vi "NEO Sensor Fault detection.vi"() -> (0 "Array":string[](array[string]), 1 "Cascade Sensor":bool, 2 "Rhino Sensors":bool, 3 "Drivebase Sensors":bool)   [LabVIEW 2018]
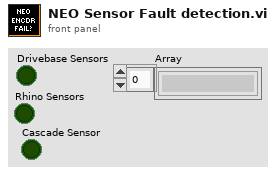
[diagram p1: front panel]
types:
  T1 = typedef "WPI_MotorControlDeviceRef.ctl" = cluster{"DeviceStatus":errorcluster, "Type":T2, "PWM":cluster{"PWM Channel":T3, "DeadBand":T4}, "CAN":cluster{"Device Number":u8, "SetOutput VI Ref":variant, "GetOutput VI Ref":variant, "Enable VI Ref":variant, "Disable VI Ref":variant, "Data":variant}, "Invert":bool, "DIO PWM":cluster{"PWM \"Enable\" Channel":T3, "DIOChannel":T5, "PWM Rate":dbl}}
  T2 = typedef "WPI_MotorControlType.ctl" = enum16{"PWM", "CAN", "DIO PWM"}
  T3 = typedef "FPGA_DIOPWMChannel.ctl" = enum8{"PWM 0", "PWM 1", "PWM 2", "PWM 3", "PWM 4", "PWM 5", "PWM 6", "PWM 7", "PWM 8", "PWM 9", "PWM MXP 0", "PWM MXP 1", "PWM MXP 2", "PWM MXP 3", "PWM MXP 4", "PWM MXP 5", "PWM MXP 6", "PWM MXP 7", "PWM MXP 8", "PWM MXP 9", "Invalid"}
  T4 = typedef "WPI_PWMDeadband.ctl" = cluster{"Name":string, "maxPositivePwm":i32, "minPositivePwm":i32, "centerPwm":i32, "maxNegativePwm":i32, "minNegativePwm":i32, "angularRange":u16}
  T5 = typedef "FPGA_DIOChannel.ctl" = enum8{"DIO 0", "DIO 1", "DIO 2", "DIO 3", "DIO 4", "DIO 5", "DIO 6", "DIO 7", "DIO 8", "DIO 9", "DIO MXP 0", "DIO MXP 1", "DIO MXP 2", "DIO MXP 3", "DIO MXP 4", "DIO MXP 5", "DIO MXP 6", "DIO MXP 7", "DIO MXP 8", "DIO MXP 9", "DIO MXP 10", "DIO MXP 11", "DIO MXP 12", "DIO MXP 13", "DIO MXP 14", "DIO MXP 15", "SPI Port CS1", "SPI Port CS2", "SPI Port CS3", "SPI Port MISO", "SPI Port MOSI", "Invalid"}
  T6 = typedef "Spark MAX Faults.ctl" = cluster{"Hard Limit Rev":bool, "Hard Limit Fwd":bool, "Soft Limit Fwd":bool, "Soft Limit Rev":bool, "Other Fault":bool, "DRV Fault":bool, "Has Reset?":bool, "CAN RX":bool, "CAN TX":bool, "EEPROM CRC":bool, "Stall":bool, "Sensor Fault":bool, "Motor Type Fault":bool, "IWDT Reset":bool, "Over Current":bool, "Brownout":bool}
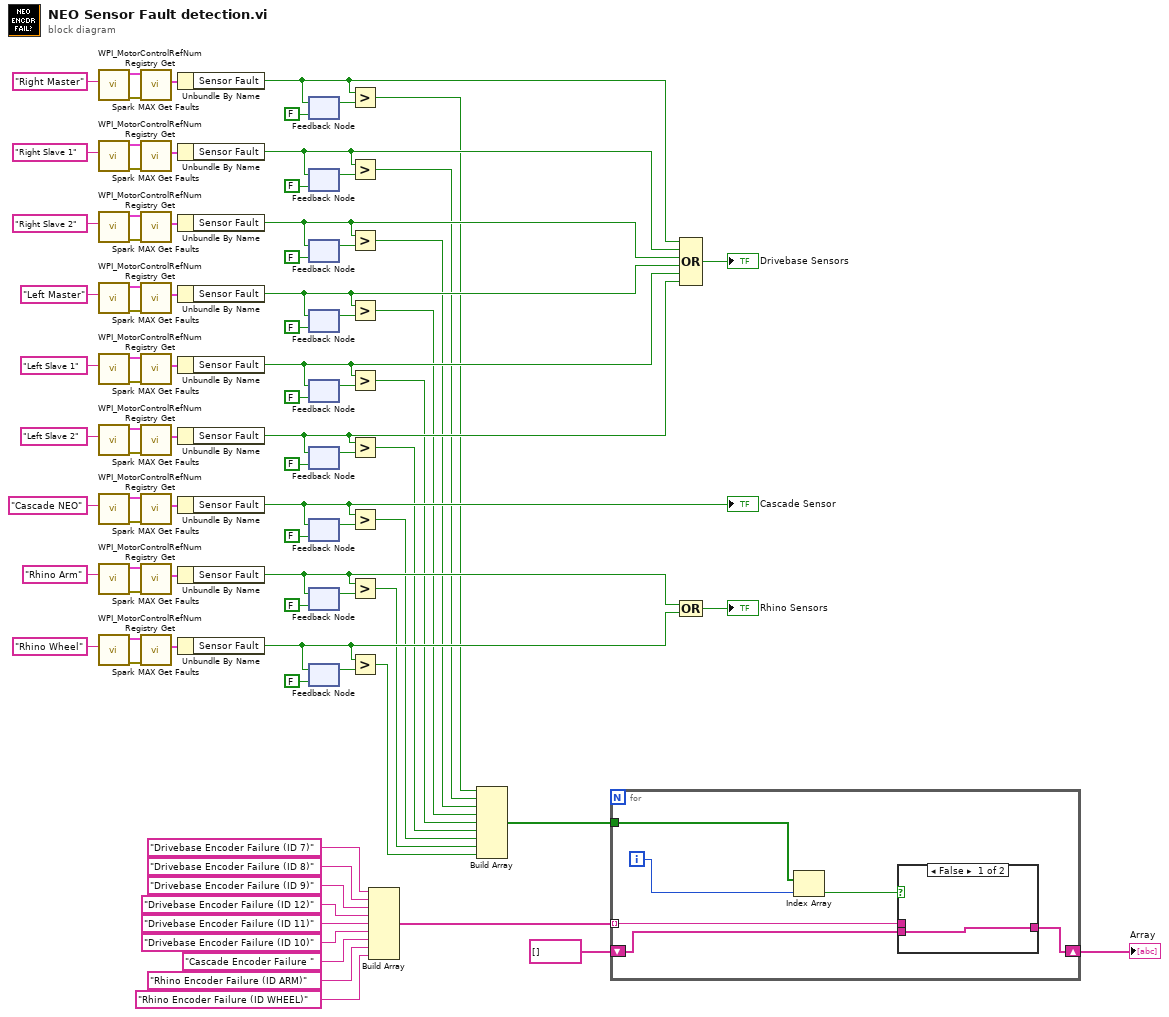
[diagram p0: block diagram]
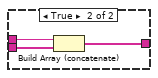
[diagram p2: hidden frame]
diagram:
  n1 = call <vilib>:"WPI_MotorControlRefNum Registry Get.vi"("refnum name"="Right Master") -> ("error out"=w75:errorcluster, "MotorControlDevRef"=w81:T1)  [unwired: 9 in]
  n2 = call <vilib>:"WPI_MotorControlRefNum Registry Get.vi"("refnum name"="Right Slave 1") -> ("error out"=w74:errorcluster, "MotorControlDevRef"=w80:T1)  [unwired: 9 in]
  n3 = call <vilib>:"WPI_MotorControlRefNum Registry Get.vi"("refnum name"="Right Slave 2") -> ("error out"=w73:errorcluster, "MotorControlDevRef"=w79:T1)  [unwired: 9 in]
  n4 = call <vilib>:"WPI_MotorControlRefNum Registry Get.vi"("refnum name"="Left Master") -> ("error out"=w72:errorcluster, "MotorControlDevRef"=w78:T1)  [unwired: 9 in]
  n5 = call <vilib>:"WPI_MotorControlRefNum Registry Get.vi"("refnum name"="Left Slave 1") -> ("error out"=w71:errorcluster, "MotorControlDevRef"=w77:T1)  [unwired: 9 in]
  n6 = call <vilib>:"WPI_MotorControlRefNum Registry Get.vi"("refnum name"="Left Slave 2") -> ("error out"=w70:errorcluster, "MotorControlDevRef"=w76:T1)  [unwired: 9 in]
  n7 = call <vilib>:"WPI_MotorControlRefNum Registry Get.vi"("refnum name"="Cascade NEO") -> ("error out"=w61:errorcluster, "MotorControlDevRef"=w60:T1)  [unwired: 9 in]
  n8 = call <vilib>:"WPI_MotorControlRefNum Registry Get.vi"("refnum name"="Rhino Arm") -> ("error out"=w55:errorcluster, "MotorControlDevRef"=w53:T1)  [unwired: 9 in]
  n9 = call <vilib>:"WPI_MotorControlRefNum Registry Get.vi"("refnum name"="Rhino Wheel") -> ("error out"=w56:errorcluster, "MotorControlDevRef"=w54:T1)  [unwired: 9 in]
  n10 = call <vilib>:"Spark MAX Get Faults.vi"("error in (no error)"=w75, "MotorControlDevRef in"=w81) -> ("Faults"=w69:T6)  [unwired: 6 in, 3 out]
  n11 = call <vilib>:"Spark MAX Get Faults.vi"("error in (no error)"=w74, "MotorControlDevRef in"=w80) -> ("Faults"=w68:T6)  [unwired: 6 in, 3 out]
  n12 = call <vilib>:"Spark MAX Get Faults.vi"("error in (no error)"=w73, "MotorControlDevRef in"=w79) -> ("Faults"=w67:T6)  [unwired: 6 in, 3 out]
  n13 = call <vilib>:"Spark MAX Get Faults.vi"("error in (no error)"=w72, "MotorControlDevRef in"=w78) -> ("Faults"=w66:T6)  [unwired: 6 in, 3 out]
  n14 = call <vilib>:"Spark MAX Get Faults.vi"("error in (no error)"=w71, "MotorControlDevRef in"=w77) -> ("Faults"=w65:T6)  [unwired: 6 in, 3 out]
  n15 = call <vilib>:"Spark MAX Get Faults.vi"("error in (no error)"=w70, "MotorControlDevRef in"=w76) -> ("Faults"=w64:T6)  [unwired: 6 in, 3 out]
  n16 = call <vilib>:"Spark MAX Get Faults.vi"("error in (no error)"=w61, "MotorControlDevRef in"=w60) -> ("Faults"=w62:T6)  [unwired: 6 in, 3 out]
  n17 = call <vilib>:"Spark MAX Get Faults.vi"("error in (no error)"=w55, "MotorControlDevRef in"=w53) -> ("Faults"=w57:T6)  [unwired: 6 in, 3 out]
  n18 = call <vilib>:"Spark MAX Get Faults.vi"("error in (no error)"=w56, "MotorControlDevRef in"=w54) -> ("Faults"=w58:T6)  [unwired: 6 in, 3 out]
  n19 = Unbundle By Name(w69) -> ("Sensor Fault"=w48:bool)
  n20 = Unbundle By Name(w68) -> ("Sensor Fault"=w30:bool)
  n21 = Unbundle By Name(w67) -> ("Sensor Fault"=w29:bool)
  n22 = Unbundle By Name(w66) -> ("Sensor Fault"=w28:bool)
  n23 = Unbundle By Name(w65) -> ("Sensor Fault"=w27:bool)
  n24 = Unbundle By Name(w64) -> ("Sensor Fault"=w26:bool)
  n25 = Unbundle By Name(w62) -> ("Sensor Fault"=w25:bool)
  "Cascade Sensor" <- w25
  n26 = Unbundle By Name(w57) -> ("Sensor Fault"=w24:bool)
  n27 = Unbundle By Name(w58) -> ("Sensor Fault"=w23:bool)
  n28 = feedback-in #1(w48) -> ()
  n29 = feedback #1(FALSE ("Sensor Fault")) -> (w49:bool)
  n30 = feedback #2(FALSE ("Sensor Fault")) -> (w45:bool)
  n31 = feedback-in #2(w30) -> ()
  n32 = feedback #3(FALSE ("Sensor Fault")) -> (w44:bool)
  n33 = feedback-in #3(w29) -> ()
  n34 = feedback #4(FALSE ("Sensor Fault")) -> (w41:bool)
  n35 = feedback-in #4(w28) -> ()
  n36 = feedback #5(FALSE ("Sensor Fault")) -> (w40:bool)
  n37 = feedback-in #5(w27) -> ()
  n38 = feedback #6(FALSE ("Sensor Fault")) -> (w37:bool)
  n39 = feedback-in #6(w26) -> ()
  n40 = feedback #7(FALSE ("Sensor Fault")) -> (w36:bool)
  n41 = feedback-in #7(w25) -> ()
  n42 = feedback #8(FALSE ("Sensor Fault")) -> (w33:bool)
  n43 = feedback-in #8(w24) -> ()
  n44 = feedback #9(FALSE ("Sensor Fault")) -> (w32:bool)
  n45 = feedback-in #9(w23) -> ()
  n46 = Greater?(x=w48, y=w49) -> (0:w22:bool)
  n47 = Greater?(x=w30, y=w45) -> (0:w21:bool)
  n48 = Greater?(x=w29, y=w44) -> (0:w20:bool)
  n49 = Greater?(x=w28, y=w41) -> (0:w19:bool)
  n50 = Greater?(x=w27, y=w40) -> (0:w18:bool)
  n51 = Greater?(x=w26, y=w37) -> (0:w17:bool)
  n52 = Greater?(x=w25, y=w36) -> (0:w16:bool)
  n53 = Greater?(x=w24, y=w33) -> (0:w15:bool)
  n54 = Greater?(x=w23, y=w32) -> (0:w14:bool)
  n55 = Build Array("Drivebase Encoder Failure (ID 7)" ("refnum name"), "Drivebase Encoder Failure (ID 8)" ("refnum name"), "Drivebase Encoder Failure (ID 9)" ("refnum name"), "Drivebase Encoder Failure (ID 12)" ("refnum name"), "Drivebase Encoder Failure (ID 11)" ("refnum name"), "Drivebase Encoder Failure (ID 10)" ("refnum name"), "Cascade Encoder Failure " ("refnum name"), "Rhino Encoder Failure (ID ARM)" ("refnum name"), "Rhino Encoder Failure (ID WHEEL)" ("refnum name")) -> (w3:string[])
  n56 = Build Array(w22, w21, w20, w19, w18, w17, w16, w15, w14) -> (w13:bool[])
  n57 = for {
    tunnel: w13 -> [w89]
    tunnel: w3 -> [w91] mode=indexing
    shift-right: [w90] -> w1
    shift-left: string[] [] -> [w92]
    i -> [w93]
    n58 = Index Array(array=w89, index=w93) -> (element=w88:bool)
    n59 = case shown="False" w88 {
      tunnel: w92 -> [w94 w97]
      tunnel: w91 -> [_ w96]
      tunnel: [w94 w95] -> w90
      frame False {
      }
      frame True {
        n60 = Build Array (concatenate)(w96, w97) -> (w95:string[])
      }
    }
  }
  "Array" <- w1
  n61 = Compound Arithmetic op=OR(w48, w30, w29, w28, w27, w26) -> (→"Drivebase Sensors":bool)
  n62 = Compound Arithmetic op=OR(w24, w23) -> (→"Rhino Sensors":bool)
